vi "ArmGetPositionPiece.vi"() -> (2 "Position":T1=enum."Middle", 3 "Game Piece":T2)   [LabVIEW 2023]
uses:
  ArmGamePiecePreset.ctl
  ArmPositionPreset.ctl
  ArmGlobal.vi
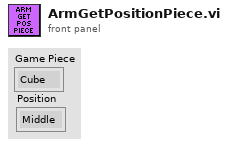
[diagram p1: front panel]
types:
  T1 = typedef "ArmPositionPreset.ctl" = enum16{"Upper", "Lower", "Middle", "Home", "Shelf", "Floor", "HalfFloor", "HalfHome"}
  T2 = typedef "ArmGamePiecePreset.ctl" = enum16{"Cube", "Cone"}
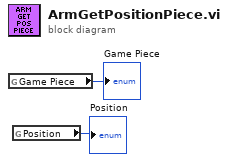
[diagram p0: block diagram]
diagram:
  n1 = global read "ArmGlobal.vi" "Game Piece"() -> (→"Game Piece":T2)
  n2 = global read "ArmGlobal.vi" "Position"() -> (→"Position":T1)
